vi "Digital Write Square Wave.vi"(7 "Duration (ms)":u32, 8 "Error In":errorcluster, 9 "Frequency (Hz)":u32, 10 "Channel":u8, 11 "LINX Resource":T1) -> (0 "Error Out":errorcluster, 3 "LINX Resource":T1)   [LabVIEW 2019, in "LMH-LINX.lvlib"]
doc: "Generate a square wave with the specified frequency for the specified duration. myRIO uses PWM channels for this function while most other devices use a DO channels.\n\nUse a duration of 0 to generate output indefinatly.\n\nUse a frequency of 0 to stop generating output."
uses:
  <vilib>/MakerHub/LINX/LMH-LINX.lvlib
  <vilib>/MakerHub/LINX/Private/Type Defs/LINX Ref.ctl
  <vilib>/MakerHub/LINX/Private/Type Defs/Platform.ctl
  <vilib>/MakerHub/LINX/Private/Type Defs/Interface.ctl
  <vilib>/MakerHub/LINX/Private/Device/Type Defs/LINX Device Config.ctl
  <vilib>/MakerHub/LINX/Private/Device/Type Defs/TCP Config.ctl
  <vilib>/MakerHub/LINX/Private/Device/Type Defs/Channels.ctl
  <vilib>/MakerHub/LINX/Private/Type Defs/Peripheral.ctl
  <vilib>/MakerHub/LINX/Private/Type Defs/Error Type.ctl
  <vilib>/MakerHub/LINX/Private/Device/Device.lvlib
  <vilib>/MakerHub/LINX/Private/myRIO/myRIO.lvlib
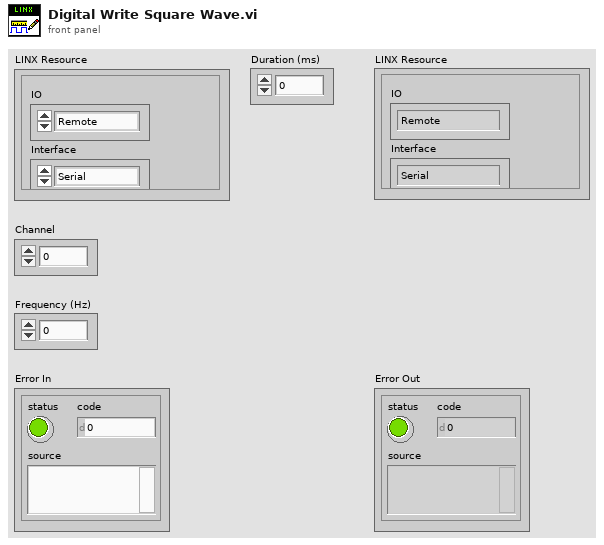
[diagram p1: front panel]
types:
  T1 = typedef "LMH-LINX.lvlib/LINX Ref.ctl" = cluster{"IO":T2, "Interface":T3, "LINX Device Config":T4}
  T2 = typedef "LMH-LINX.lvlib/Platform.ctl" = enum16{"Remote", "Local"}
  T3 = typedef "LMH-LINX.lvlib/Interface.ctl" = enum16{"Serial", "TCP"}
  T4 = typedef "LMH-LINX.lvlib/Device.lvlib/LINX Device Config.ctl" = cluster{"Interface":T3, "COM Port":refnum<visa-resource-name>, "TCP Configuration":T5, "Device Family":u8, "Device ID":u8, "Device Name":string, "TCP Ref":refnum<k5>, "Channels":T6}
  T5 = typedef "LMH-LINX.lvlib/Device.lvlib/TCP Config.ctl" = cluster{"IP Address":string, "Port":u16}
  T6 = typedef "LMH-LINX.lvlib/Channels.ctl" = cluster{"DI":u8[], "DO":u8[], "AI":u8[], "AO":u8[], "PWM":u8[], "QE":u8[], "UART":u8[], "I2C 2":u8[], "SPI":u8[], "CAN":u8[], "Servo":u8[], "AI Ref (V)":dbl, "AI Resolution (Bits)":u8, "AO Ref (V)":dbl, "AO Resolution (Bits)":u8}
  T7 = typedef "LMH-LINX.lvlib/Peripheral.ctl" = enum8{"DI", "DO", "AI", "AO", "PWM", "QE", "UART", "I2C", "SPI", "CAN", "Servo"}
  T8 = typedef "LMH-LINX.lvlib/Error Type.ctl" = enum16{"Unknown", "Timeout", "Corrupt Return Packet", "Unable To Connect", "Command Not Supported", "Channel DNE", "Invalid COM Config", "Firmware Version Mismatch", "myRIO Support", "CMD Specific Error", "Local IO Not Supported"}
  T9 = typedef "PWM.lvlib/PWM Reference.ctl" = cluster{"myRIO Reference":T10, "PWM Channels Enum":T14, "PWM Configuration":T15}
  T10 = typedef "myRIO Generic Hardware Reference.ctl" = cluster{"myRIO Model":T11, "myRIO Hardware Reference":T12}
  T11 = typedef "Hardware Version Enum.ctl" = enum16{"Unknown", "myRIO-1900", "myRIO-1950"}
  T12 = typedef "myRIO v1.0 Reference.ctl" = cluster{"Generic FPGA Reference":T13, "Allow multiple opens":bool}
  T13 = typedef "Generic FPGA Reference.ctl" = refnum<k20>
  T14 = typedef "PWM Channels Enum.ctl" = enum16{"Not Connected", "C/PWM0", "C/PWM1", "A/PWM0", "A/PWM1", "A/PWM2", "B/PWM0", "B/PWM1", "B/PWM2"}
  T15 = typedef "PWM.lvlib/PWM Configuration.ctl" = cluster{"Frequency":dbl, "Duty Cycle":dbl}
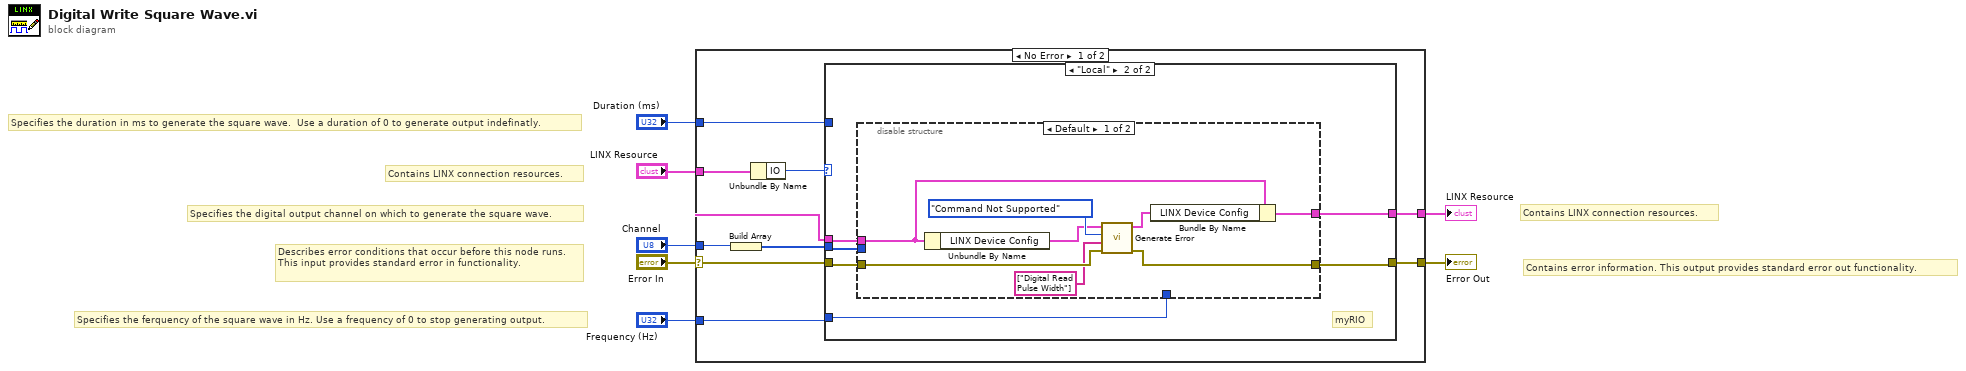
[diagram p0: block diagram]
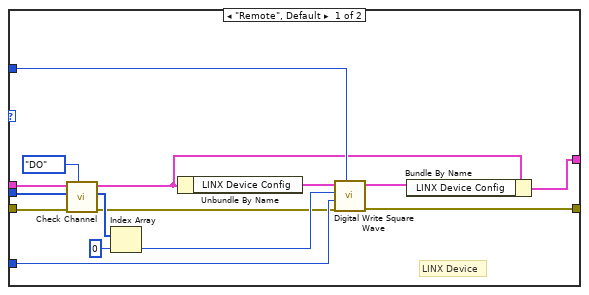
[diagram p2: hidden frame]
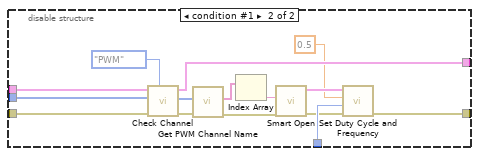
[diagram p3: hidden frame]
diagram:
  # "Specifies the ferquency of the square wave in Hz. Use a frequency of 0 to stop generating output."
  # "Specifies the digital output channel on which to generate the square wave."
  # "Specifies the duration in ms to generate the square wave.  Use a duration of 0 to generate output indefinatly."
  # "Contains LINX connection resources."
  # "Contains error information. This output provides standard error out functionality."
  # "Contains LINX connection resources."
  # "Describes error conditions that occur before this node runs. This input provides standard error in functionality."
  n1 = case shown="No Error" "Error In" {
    selector: "Error In" -> [w8 w62]
    tunnel: [w15 w62] -> w7
    tunnel: [w14 w61] -> w6
    tunnel: "Channel" -> [w13 _]
    tunnel: "Duration (ms)" -> [w12 _]
    tunnel: "Frequency (Hz)" -> [w11 _]
    tunnel: "LINX Resource" -> [w9 w61]
    frame No Error {
      n2 = Build Array(w13) -> (w10:u8[])
      n3 = Unbundle By Name(w9) -> ("IO"=w16:T2)
      n4 = case shown="\"Local\"" w16 {
        tunnel: w8 -> [w23 w37]
        tunnel: w9 -> [w20 w36]
        tunnel: [w27 w32] -> w15
        tunnel: [w31 w34] -> w14
        tunnel: w10 -> [w18 w35]
        tunnel: w12 -> [w24 _]
        tunnel: w11 -> [w25 w33]
        frame "Remote", Default {
          # "LINX Device"
          n5 = call <vilib>:"Check Channel.vi"("Peripheral"=Peripheral."DO", "Error In"=w23, "Channels"=w18, "LINX Resource"=w20) -> ("Error Out"=w21:errorcluster, "Channels"=w22:u8[], "LINX Resource"=w19:T1)  [unwired: 5 in]
          n6 = Index Array(array=w22, index=0) -> (element=w26:u8)
          n7 = Unbundle By Name(w19) -> ("LINX Device Config"=w29:T4)
          n8 = call <vilib>:"Digital Write Square Wave.vi"("Duration (ms)"=w24, "Error In"=w21, "Frequency"=w25, "DO Channel"=w26, "LINX Device Config"=w29) -> ("Error Out"=w27:errorcluster, "LINX Device Config"=w28:T4)  [unwired: 5 in]
          n9 = Bundle By Name(cluster=w19, "LINX Device Config"=w28) -> (w31:T1)
        }
        frame "Local" {
          # "myRIO"
          n10 = disable-structure shown="Default" {
            disable-tunnel: w37 -> [w41 w60]
            disable-tunnel: w36 -> [w42 w59]
            disable-tunnel: w35 -> [_ w58]
            disable-tunnel: [w38 w57] -> w34
            disable-tunnel: w33 -> [_ w56]
            disable-tunnel: [w40 w55] -> w32
            frame condition #0 (active) {
              n11 = Unbundle By Name(w42) -> ("LINX Device Config"=w44:T4)
              n12 = call <vilib>:"Generate Error.vi"("Error In"=w41, "Arguments"=string[] ["Digital Read Pulse Width"], "Error Type"=Error_Type."Command Not Supported", "LINX Device Config"=w44) -> ("Error Out"=w40:errorcluster, "Dup LINX Device Config"=w43:T4)  [unwired: 6 in]
              n13 = Bundle By Name(cluster=w42, "LINX Device Config"=w43) -> (w38:T1)
            }
            frame condition #1 {
              n14 = call <vilib>:"Check Channel.vi"("Peripheral"=Peripheral."PWM", "Error In"=w60, "Channels"=w58, "LINX Resource"=w59) -> ("Error Out"=w53:errorcluster, "Channels"=w54:u8[], "LINX Resource"=w57:T1)  [unwired: 5 in]
              n15 = call <vilib>:"Get PWM Channel Name.vi"("Error In"=w53, "PWM Channel Nums"=w54) -> ("Error Out"=w49:errorcluster, "PWM Channels"=w48:string[])  [unwired: 8 in]
              n16 = Index Array(array=w48) -> (element=w47:string)  [unwired: 1 in]
              n17 = call <vilib>:"Smart Open.vi"("error in (no error)"=w49, "Channel Name"=w47) -> ("error out"=w50:errorcluster, "PWM Ref Out"=w51:T9)  [unwired: 8 in]
              n18 = call <vilib>:"Set Duty Cycle and Frequency.vi"("error in (no error)"=w50, "Frequency [Hz]"=w56, "Duty Cycle"=0.5 ("Duty Cycle (0-1)"), "PWM Ref In"=w51) -> ("error out"=w55:errorcluster)  [unwired: 5 in, 1 out]
            }
          }
        }
      }
    }
    frame Error {
    }
  }
  "Error Out" <- w7
  "LINX Resource" <- w6
